vi "23384_Davis_Poku_Amankwa_Amankwa.DavisPoku.MNE1201.3.3_348255_202539885.vi"() -> ()   [LabVIEW 2018]
panel:
  out "?":cluster{dbl, dbl, dbl[]}(graph)
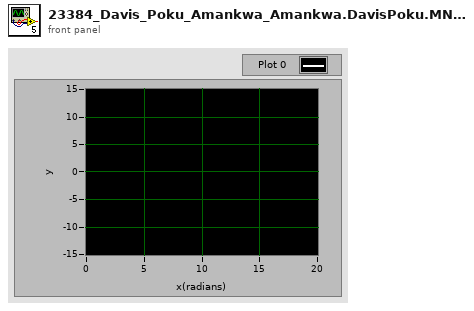
[diagram p1: front panel]
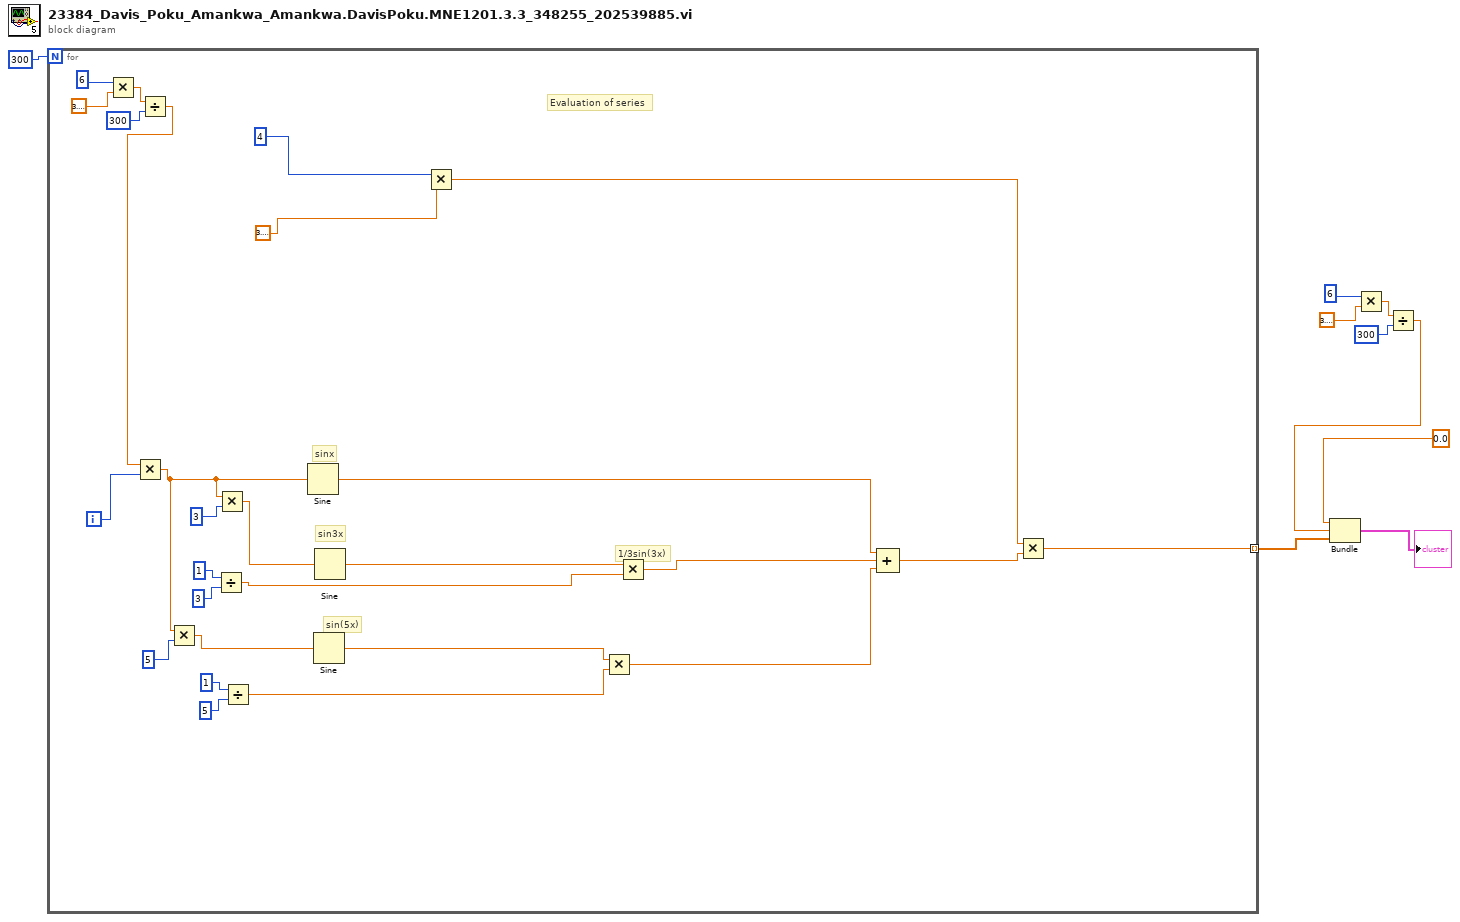
[diagram p0: block diagram]
diagram:
  n1 = for {
    N: 300 -> [_]
    tunnel: [w10] -> w7 mode=indexing
    i -> [w36]
    # "sin(5x)"
    # "1/3sin(3x)"
    # "sin3x"
    # "sinx"
    # "Evaluation of series"
    n2 = Multiply(x=6, y=3.141592653589793) -> (x*y=w35:dbl)
    n3 = Divide(x=w35, y=300) -> (x/y=w31:dbl)
    n4 = Multiply(x=w31, y=w36) -> (x*y=w18:dbl)
    n5 = Multiply(x=w18, y=5) -> (x*y=w16:dbl)
    n6 = Divide(x=1, y=3) -> (x/y=w24:dbl)
    n7 = Multiply(x=w18, y=3) -> (x*y=w27:dbl)
    n8 = Divide(x=1, y=5) -> (x/y=w20:dbl)
    n9 = Sine(x=w18) -> (sin(x)=w13:dbl)
    n10 = Sine(x=w16) -> (sin(x)=w19:dbl)
    n11 = Sine(x=w27) -> (sin(x)=w23:dbl)
    n12 = Multiply(x=4, y=3.141592653589793) -> (x*y=w12:dbl)
    n13 = Multiply(x=w19, y=w20) -> (x*y=w15:dbl)
    n14 = Multiply(x=w23, y=w24) -> (x*y=w14:dbl)
    n15 = Compound Arithmetic op=ADD(w13, w14, w15) -> (w11:dbl)
    n16 = Multiply(x=w12, y=w11) -> (x*y=w10:dbl)
  }
  n17 = Multiply(x=6, y=3.141592653589793) -> (x*y=w5:dbl)
  n18 = Divide(x=w5, y=300) -> (x/y=w1:dbl)
  n19 = Bundle(0.0, w1, w7) -> (→"?":cluster{dbl, dbl, dbl[]})  [unwired: 1 in]
